vi "Falha.vi"() -> ()   [LabVIEW 2018]
uses:
  Global_Telescopio.vi
panel:
  out "String":string="\n\n\nATENÇÃO: Falha de Comunicação\nEntre em contato com o técnico plantonista"
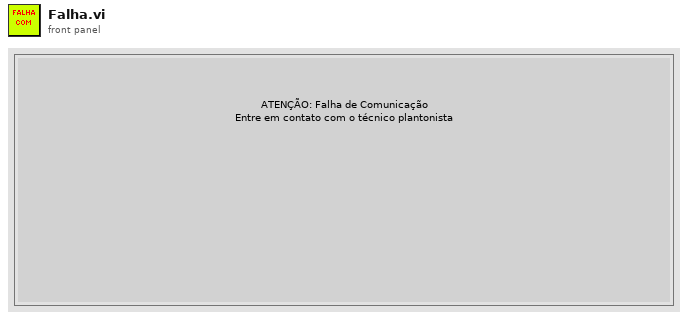
[diagram p1: front panel]
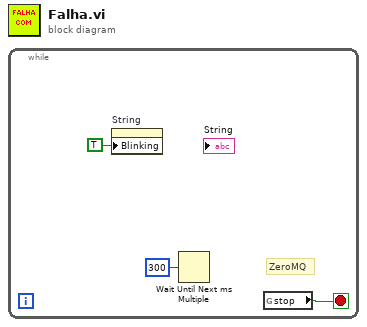
[diagram p0: block diagram]
diagram:
  n1 = while {
    stop <- w1 stop-if-true
    # "ZeroMQ"
    n2 = property on="String" class="Str"("Blinking"=TRUE) -> ()  [unwired: 2 in, 2 out]
    n3 = Wait Until Next ms Multiple(millisecond multiple=u32 300) -> ()  [unwired: 1 out]
    n4 = global read "Global_Telescopio.vi" "stop"() -> (w1:bool)
  }
